vi "TTA_Parse_TTile_Loss.vi"(8 "error in":errorcluster, 9 "Channel":enum16{"CH0", "CH1"}(ring), 10 "Antenna":T1(ring), 11 "Working Directory":path) -> (0 "error out":errorcluster, 3 "TTile Loss (dB)":dbl)   [LabVIEW 2016]
uses:
  <vilib>/Utility/file.llb/Read Delimited Spreadsheet (string).vi
panel:
  in  "Frequency (MHz)":dbl
  out "all rows":string[][](array[string])
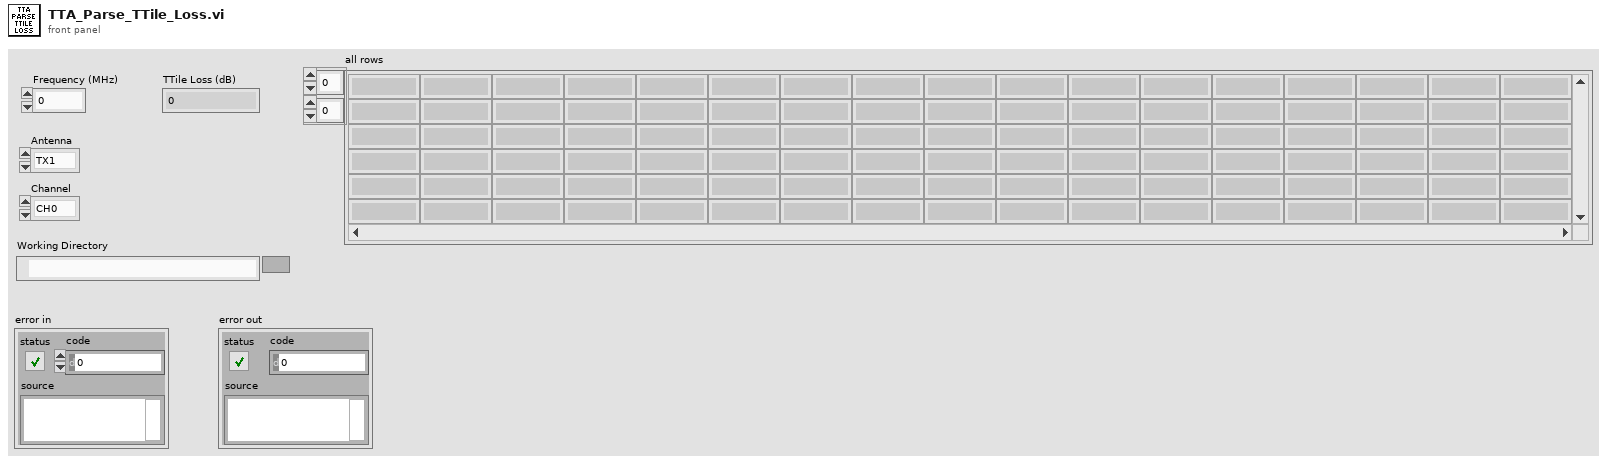
[diagram p1: front panel]
types:
  T1 = enum16{"TX1", "TX2", "TX3", "TX4", "RX1", "RX2", "RX3", "RX4"}
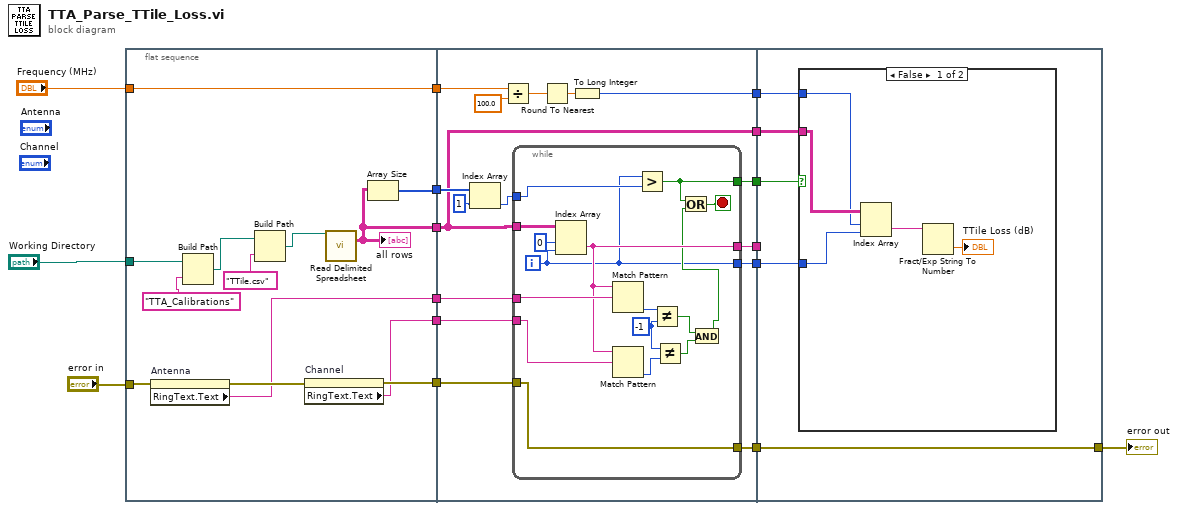
[diagram p0: block diagram]
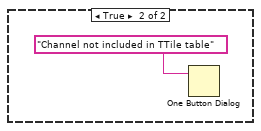
[diagram p2: hidden frame]
diagram:
  n1 = flat-sequence {
    tunnel: "error in" -> [w24]
    tunnel: "Working Directory" -> [w29]
    tunnel: "Frequency (MHz)" -> [w19]
    tunnel: [w18] -> w14
    tunnel: [w22] -> w12
    tunnel: [w21] -> w11
    tunnel: [w20] -> w10
    tunnel: [w19] -> w7
    tunnel: [w17] -> w6
    tunnel: w14 -> [w37]
    tunnel: w12 -> [w31]
    tunnel: w11 -> [w45]
    tunnel: w10 -> [w44]
    tunnel: [w43] -> w9
    tunnel: [w42] -> w8
    tunnel: w7 -> [w36]
    tunnel: w6 -> [w41]
    tunnel: [w38] -> w5
    tunnel: [w37] -> w4
    tunnel: [w32] -> w3
    tunnel: [w30] -> w2
    tunnel: w9 -> [w64]
    tunnel: w8 -> [_]
    tunnel: w5 -> [w66]
    tunnel: w4 -> [w65]
    tunnel: w3 -> [w63]
    tunnel: [w62] -> w1
    tunnel: w2 -> [w62]
    frame #0 {
      n2 = property on="Antenna" class="Enum (strict)"(error in=w24) -> (error out=w23:errorcluster, "RingText.Text"=w21:string)  [unwired: 1 in, 1 out]
      n3 = Build Path(base path=w29, name or relative path="TTA_Calibrations") -> (appended path=w26:path)
      n4 = Build Path(base path=w26, name or relative path="TTile.csv") -> (appended path=w25:path)
      n5 = property on="Channel" class="Enum (strict)"(error in=w23) -> (error out=w22:errorcluster, "RingText.Text"=w20:string)  [unwired: 1 in, 1 out]
      n6 = call-poly <vilib>:"Read Delimited Spreadsheet.vi"("file path (dialog if empty)"=w25) -> ("all rows"=w18:string[][])  [unwired: 9 in, 5 out]
      "all rows" <- w18
      n7 = Array Size(array=w18) -> (size(s)=w17:i32[])
    }
    frame #1 {
      n8 = Index Array(array=w41, index=1) -> (element=w39:i32)
      n9 = Divide(x=w36, y=100.0) -> (x/y=w34:dbl)
      n10 = while {
        tunnel: w37 -> [w61]
        tunnel: w45 -> [w59]
        tunnel: w44 -> [w58]
        tunnel: [w47] -> w43
        tunnel: [w52] -> w42
        tunnel: w39 -> [w49]
        tunnel: [w48] -> w38
        tunnel: w31 -> [w46]
        tunnel: [w46] -> w30
        i -> [w47]
        stop <- w50 stop-if-true
        w55 = -1 ("y")
        n11 = Index Array(array=w61, index (row)=0 ("disabled index (row)"), index (col)=w47) -> (element=w52:string)
        n12 = Match Pattern(string=w52, regular expression=w59) -> (offset past match=w57:i32)  [unwired: 1 in, 3 out]
        n13 = Match Pattern(string=w52, regular expression=w58) -> (offset past match=w56:i32)  [unwired: 1 in, 3 out]
        n14 = Greater?(x=w47, y=w49) -> (0:w48:bool)
        n15 = Not Equal?(x=w57, y=w55) -> (x != y?=w54:bool)
        n16 = Not Equal?(x=w55, y=w56) -> (x != y?=w53:bool)
        n17 = And(x=w54, y=w53) -> (x .and. y?=w51:bool)
        n18 = Or(x=w48, y=w51) -> (x .or. y?=w50:bool)
      }
      n19 = Round To Nearest(number=w34) -> (nearest integer value=w33:dbl)
      n20 = To Long Integer(number=w33) -> (32bit integer=w32:i32)
    }
    frame #2 {
      n21 = case shown="False" w66 {
        tunnel: w65 -> [w71 _]
        tunnel: w64 -> [w69 _]
        tunnel: w63 -> [w70 _]
        frame False {
          n22 = Index Array(array=w71, index (row)=w70, index (col)=w69) -> (element=w68:string)
          n23 = Fract/Exp String To Number(string=w68) -> (number=→"TTile Loss (dB)":dbl)  [unwired: 3 in, 1 out]
        }
        frame True {
          n24 = One Button Dialog(message="Channel not included in TTile table") -> ()  [unwired: 1 in, 1 out]
        }
      }
    }
  }
  "error out" <- w1
